vi "Script_Import.vi"(8 "error in (no error)":errorcluster, 11 "Seq":T1[](array[typedef])) -> (0 "error out":errorcluster)   [LabVIEW 2016, in "SeqProcessor.lvlib"]
uses:
  SeqProcessor.lvlib
  controls/StepScript.ctl
  controls/StepType.ctl
  controls/Step.ctl
  controls/NormalStep.ctl
  controls/StepAction.ctl
  controls/StepResult.ctl
  controls/StepStatus.ctl
  controls/JumpStep.ctl
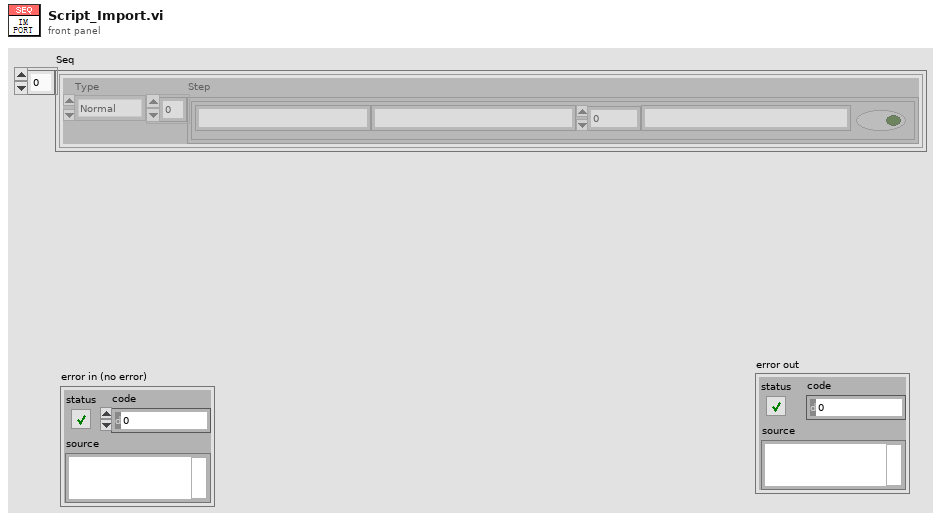
[diagram p1: front panel]
types:
  T1 = typedef "SeqProcessor.lvlib/StepScript.ctl" = cluster{"Type":T2, "Step":cluster{"Action":string, "Process":string, "Jump":i32, "Data":string, "Condition":bool}[]}
  T2 = typedef "SeqProcessor.lvlib/StepType.ctl" = enum16{"Normal", "Parallel", "Conditional", "Jump"}
  T3 = typedef "SeqProcessor.lvlib/Step.ctl" = cluster{"Type":T2, "Step":variant}
  T4 = typedef "SeqProcessor.lvlib/StepAction.ctl" = cluster{"Action":string, "Process":string, "Data":variant, "Condition":variant}
  T5 = typedef "SeqProcessor.lvlib/NormalStep.ctl" = cluster{"Action":T4, "Result":T6}
  T6 = typedef "SeqProcessor.lvlib/StepResult.ctl" = cluster{"Status":T7, "Message":string, "Data":variant}
  T7 = typedef "SeqProcessor.lvlib/StepStatus.ctl" = enum16{"Undone", "Finish", "Error"}
  T8 = typedef "SeqProcessor.lvlib/JumpStep.ctl" = cluster{"Action":T4, "Jump":i32, "Result":T6}
  T9 = cluster{"Action":string, "Process":string, "Jump":i32, "Data":string, "Condition":bool}[]
  T10 = cluster{"Action":string, "Process":string, "Jump":i32, "Data":string, "Condition":bool}
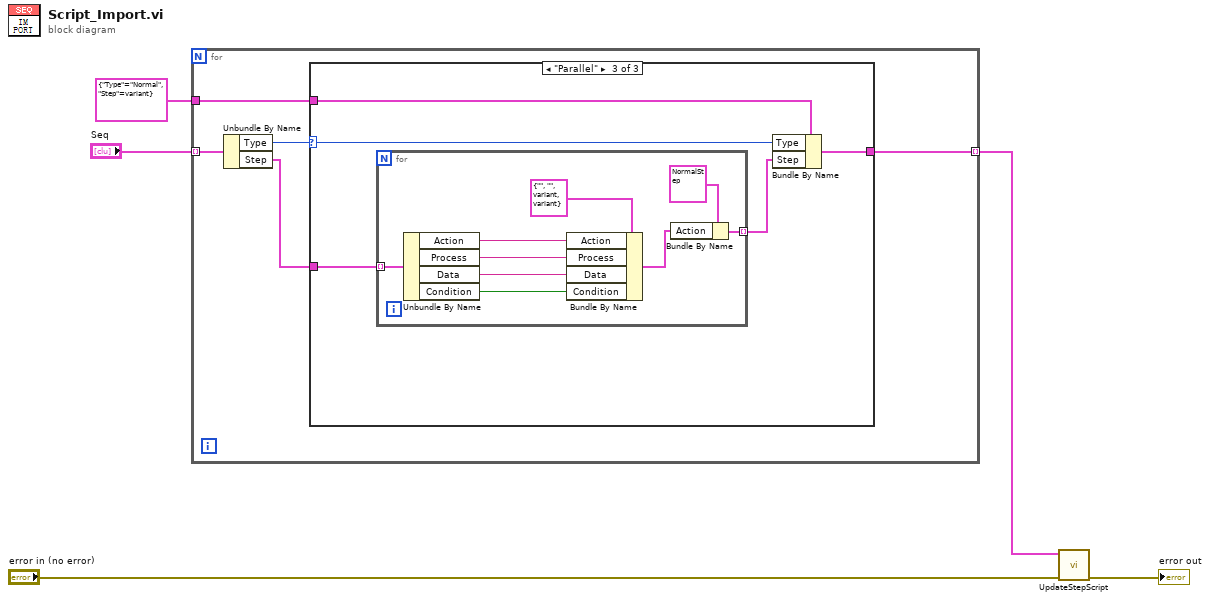
[diagram p0: block diagram]
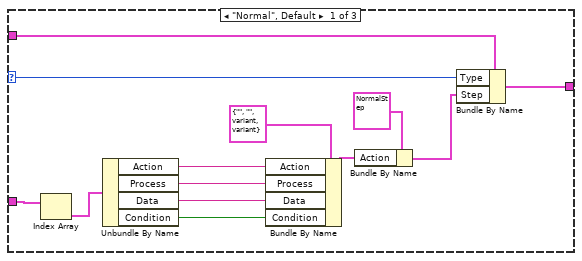
[diagram p2: hidden frame]
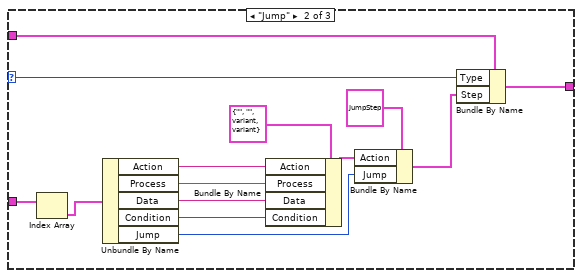
[diagram p3: hidden frame]
diagram:
  n1 = for {
    tunnel: T3 {"Type"=enum."Normal", "Step"=variant} ("Step") -> [w9]
    tunnel: "Seq" -> [w7] mode=indexing
    tunnel: [w8] -> w2 mode=indexing
    n2 = Unbundle By Name(w7) -> ("Type"=w10:T2, "Step"=w6:T9)
    n3 = case shown="\"Parallel\"" w10 {
      selector: w10 -> [w21 w36 w40]
      tunnel: w6 -> [w12 w25 w42]
      tunnel: w9 -> [w22 w37 w41]
      tunnel: [w20 w35 w39] -> w8
      frame "Normal", Default {
        n4 = Index Array(array=w12) -> (element=w11:T10)  [unwired: 1 in]
        n5 = Unbundle By Name(w11) -> ("Action"=w16:string, "Process"=w15:string, "Data"=w14:string, "Condition"=w13:bool)
        n6 = Bundle By Name(cluster=T4 {"Action"="", "Process"="", "Data"=variant, "Condition"=variant} ("Action"), "Action"=w16, "Process"=w15, "Data"=w14, "Condition"=w13) -> (w17:T4)
        n7 = Bundle By Name(cluster=T5 {"Action"={"Action"="", "Process"="", "Data"=variant, "Condition"=variant(bool FALSE)}, "Result"={"Status"=enum."Undone", "Message"="", "Data"=variant}} ("NormalStep"), "Action"=w17) -> (w19:T5)
        n8 = Bundle By Name(cluster=w22, "Type"=w21, "Step"=w19) -> (w20:T3)
      }
      frame "Jump" {
        n9 = Index Array(array=w25) -> (element=w24:T10)  [unwired: 1 in]
        n10 = Unbundle By Name(w24) -> ("Action"=w31:string, "Process"=w30:string, "Data"=w29:string, "Condition"=w28:bool, "Jump"=w26:i32)
        n11 = Bundle By Name(cluster=T4 {"Action"="", "Process"="", "Data"=variant, "Condition"=variant} ("Action"), "Action"=w31, "Process"=w30, "Data"=w29, "Condition"=w28) -> (w32:T4)
        n12 = Bundle By Name(cluster=T8 {"Action"={"Action"="", "Process"="", "Data"=variant, "Condition"=variant(bool FALSE)}, "Jump"=0, "Result"={"Status"=enum."Undone", "Message"="", "Data"=variant}} ("JumplStep"), "Action"=w32, "Jump"=w26) -> (w34:T8)
        n13 = Bundle By Name(cluster=w37, "Type"=w36, "Step"=w34) -> (w35:T3)
      }
      frame "Parallel" {
        n14 = for {
          tunnel: w42 -> [w51] mode=indexing
          tunnel: [w43] -> w38 mode=indexing
          n15 = Unbundle By Name(w51) -> ("Action"=w49:string, "Process"=w48:string, "Data"=w47:string, "Condition"=w46:bool)
          n16 = Bundle By Name(cluster=T4 {"Action"="", "Process"="", "Data"=variant, "Condition"=variant} ("Action"), "Action"=w49, "Process"=w48, "Data"=w47, "Condition"=w46) -> (w44:T4)
          n17 = Bundle By Name(cluster=T5 {"Action"={"Action"="", "Process"="", "Data"=variant, "Condition"=variant(bool FALSE)}, "Result"={"Status"=enum."Undone", "Message"="", "Data"=variant}} ("NormalStep"), "Action"=w44) -> (w43:T5)
        }
        n18 = Bundle By Name(cluster=w41, "Type"=w40, "Step"=w38) -> (w39:T3)
      }
    }
  }
  n19 = call "UpdateStepScript.vi"("error in (no error)"="error in (no error)", "StepScript"=w2) -> ("error out"=→"error out":errorcluster)  [unwired: 9 in]
